vi "EF_ReadVisualDataQ.vi"(10 "EF_GUIThread_QDataList":T1[](array[typedef]), 11 "EF_GUIThread_QData":T1) -> (0 "Error":errorcluster, 3 "EF_GUIThread_QData_out":T1, 4 "isError":bool)   [LabVIEW 2017]
uses:
  Types/EF_GUIThread_QData.ctl
  Types/EF_GUIThread_QCmds.ctl
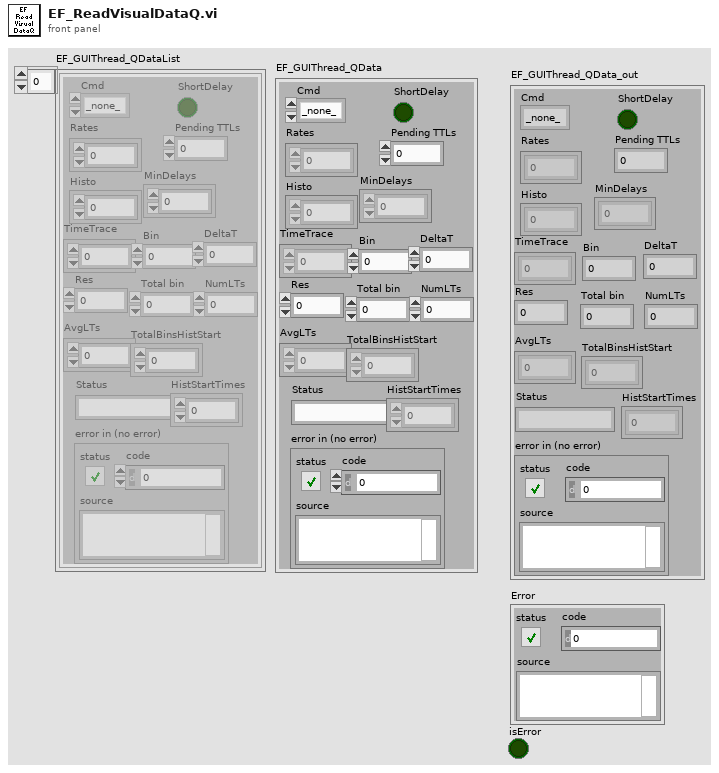
[diagram p1: front panel]
types:
  T1 = typedef "EF_GUIThread_QData.ctl" = cluster{"Histo":u32[], "Rates":i32[], "Cmd":T2, "Res":dbl, "TimeTrace":u32[], "Bin":i32, "Status":string, "Total bin":u64, "AvgLTs":dbl[], "TotalBinsHistStart":u64[], "HistStartTimes":dbl[], "MinDelays":dbl[], "ShortDelay":bool, "Pending TTLs":i32, "error in (no error)":errorcluster, "DeltaT":dbl, "NumLTs":i32}
  T2 = typedef "EF_GUIThread_QCmds.ctl" = enum16{"_none_", "Res", "Histo", "TTrace", "Lifetime", "Rates", "Status", "ShortDelay", "_Error_"}
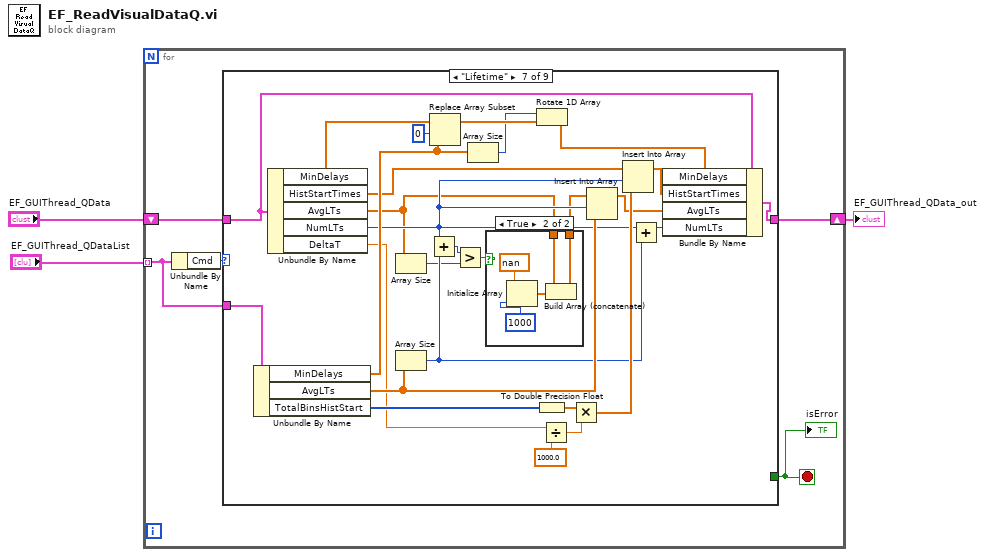
[diagram p0: block diagram]
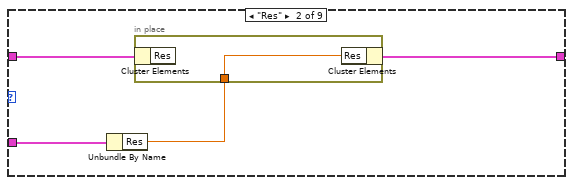
[diagram p3: hidden frame]
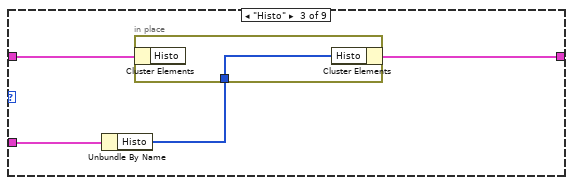
[diagram p4: hidden frame]
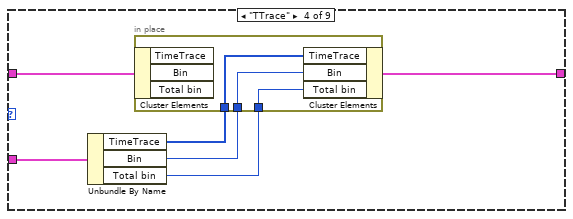
[diagram p5: hidden frame]
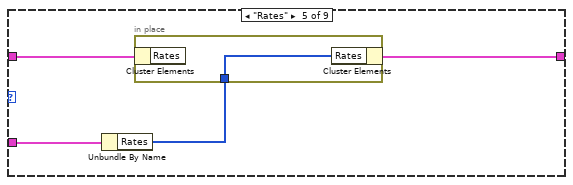
[diagram p6: hidden frame]
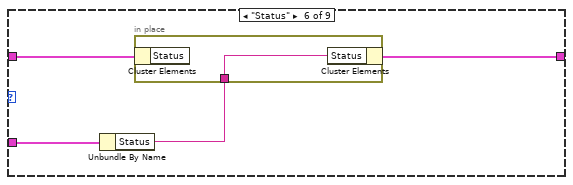
[diagram p7: hidden frame]
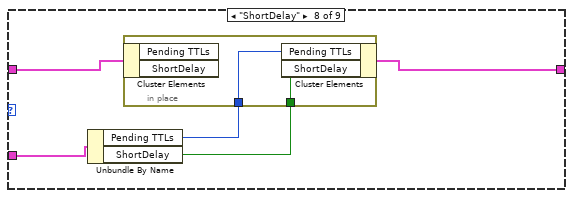
[diagram p9: hidden frame]
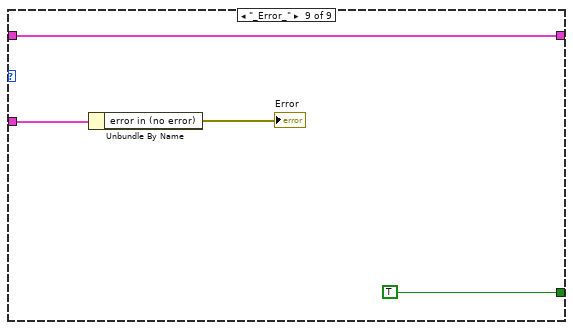
[diagram p10: hidden frame]
diagram:
  n1 = for {
    tunnel: "EF_GUIThread_QDataList" -> [w5] mode=indexing
    shift-right: [w6] -> w1
    shift-left: "EF_GUIThread_QData" -> [w7]
    stop <- w4 stop-if-true
    n2 = Unbundle By Name(w5) -> ("Cmd"=w8:T2)
    n3 = case shown="\"Lifetime\"" w8 {
      tunnel: w7 -> [w9 w13 w18 w25 w32 w37 w57 w76 w81]
      tunnel: [w9 w12 w17 w24 w31 w36 w63 w75 w81] -> w6
      tunnel: w5 -> [_ w11 w16 w23 w30 w35 w65 w74 w82]
      tunnel: [_ _ _ _ _ _ _ _ TRUE] -> w4
      frame "_none_", Default {
      }
      frame "Res" {
        n4 = Unbundle By Name(w11) -> ("Res"=w10:dbl)
        n5 = in-place {
          in-place-border: w10 -> [w14]
          n6 = in-place-cluster #1(w13) -> ()  [unwired: 1 out]
          n7 = in-place-cluster #1("Res"=w14) -> (w12:T1)
        }
      }
      frame "Histo" {
        n8 = Unbundle By Name(w16) -> ("Histo"=w15:u32[])
        n9 = in-place {
          in-place-border: w15 -> [w19]
          n10 = in-place-cluster #2(w18) -> ()  [unwired: 1 out]
          n11 = in-place-cluster #2("Histo"=w19) -> (w17:T1)
        }
      }
      frame "TTrace" {
        n12 = Unbundle By Name(w23) -> ("TimeTrace"=w22:u32[], "Bin"=w21:i32, "Total bin"=w20:u64)
        n13 = in-place {
          in-place-border: w22 -> [w28]
          in-place-border: w21 -> [w27]
          in-place-border: w20 -> [w26]
          n14 = in-place-cluster #3(w25) -> ()  [unwired: 3 out]
          n15 = in-place-cluster #3("TimeTrace"=w28, "Bin"=w27, "Total bin"=w26) -> (w24:T1)
        }
      }
      frame "Rates" {
        n16 = Unbundle By Name(w30) -> ("Rates"=w29:i32[])
        n17 = in-place {
          in-place-border: w29 -> [w33]
          n18 = in-place-cluster #4(w32) -> ()  [unwired: 1 out]
          n19 = in-place-cluster #4("Rates"=w33) -> (w31:T1)
        }
      }
      frame "Status" {
        n20 = Unbundle By Name(w35) -> ("Status"=w34:string)
        n21 = in-place {
          in-place-border: w34 -> [w38]
          n22 = in-place-cluster #5(w37) -> ()  [unwired: 1 out]
          n23 = in-place-cluster #5("Status"=w38) -> (w36:T1)
        }
      }
      frame "Lifetime" {
        n24 = Unbundle By Name(w65) -> ("MinDelays"=w58:dbl[], "AvgLTs"=w64:dbl[], "TotalBinsHistStart"=w62:u64[])
        n25 = Unbundle By Name(w57) -> ("MinDelays"=w49:dbl[], "HistStartTimes"=w46:dbl[], "AvgLTs"=w40:dbl[], "NumLTs"=w44:i32, "DeltaT"=w42:dbl)
        n26 = Array Size(array=w40) -> (size(s)=w43:i32)
        n27 = Array Size(array=w64) -> (size(s)=w55:i32)
        n28 = Add(x=w44, y=w55) -> (x+y=w54:i32)
        n29 = Replace Array Subset(array=w49, new element=w58, index=0) -> (w52:dbl[])
        n30 = Greater?(x=w54, y=w43) -> (0:w41:bool)
        n31 = Array Size(array=w58) -> (size(s)=w50:i32)
        n32 = case shown="True" w41 {
          tunnel: w40 -> [w66 w69]
          tunnel: [w66 w67] -> w39
          frame False {
          }
          frame True {
            n33 = Initialize Array(nan ("element"), 1000 ("dimension size")) -> (w68:dbl[])
            n34 = Build Array (concatenate)(w69, w68) -> (w67:dbl[])
          }
        }
        n35 = Rotate 1D Array(1:w52, 2:w50) -> (0:w51:dbl[])
        n36 = To Double Precision Float(number=w62) -> (double precision float=w61:dbl[])
        n37 = Divide(x=w42, y=1000.0) -> (x/y=w59:dbl)
        n38 = Multiply(x=w61, y=w59) -> (x*y=w56:dbl[])
        n39 = Insert Into Array(array=w39, index=w44, new element=w64) -> (w47:dbl[])
        n40 = Insert Into Array(array=w46, index=w44, new element=w56) -> (w45:dbl[])
        n41 = Add(x=w44, y=w55) -> (x+y=w48:i32)
        n42 = Bundle By Name(cluster=w57, "MinDelays"=w51, "HistStartTimes"=w45, "AvgLTs"=w47, "NumLTs"=w48) -> (w63:T1)
      }
      frame "ShortDelay" {
        n43 = Unbundle By Name(w74) -> ("Pending TTLs"=w72:i32, "ShortDelay"=w73:bool)
        n44 = in-place {
          in-place-border: w73 -> [w78]
          in-place-border: w72 -> [w77]
          n45 = in-place-cluster #6(w76) -> ()  [unwired: 2 out]
          n46 = in-place-cluster #6("Pending TTLs"=w77, "ShortDelay"=w78) -> (w75:T1)
        }
      }
      frame "_Error_" {
        n47 = Unbundle By Name(w82) -> ("error in (no error)"=→"Error":errorcluster)
      }
    }
    "isError" <- w4
  }
  "EF_GUIThread_QData_out" <- w1
